vi "read_exist_OPUS.vi"() -> ()   [LabVIEW 2010]
panel:
  in  "functionpath":path=path "D:/Research_CfA/FTS"
  out "used time":dbl
  in  "ifg_path":path=path "D:/Research_CfA/FTS/ha_20150807_ifg"
  in  "spec_path":path=path "D:/Research_CfA/FTS/ha_20150807"
  out "XY Graph 6":cluster{"spec":dbl[], "spec":dbl[]}(graph)
  out "XY Graph 5":cluster{"spec":dbl[], "spec":dbl[]}(graph)
  out "XY Graph 4":cluster{"spec":dbl[], "spec":dbl[]}(graph)
  out "XY Graph 3":cluster{"spec":dbl[], "spec":dbl[]}(graph)
  out "XY Graph 2":cluster{"spec":dbl[], "spec":dbl[]}(graph)
  out "XY Graph":cluster{"spec":dbl[], "spec":dbl[]}(graph)
  in  "observation":string="ha"
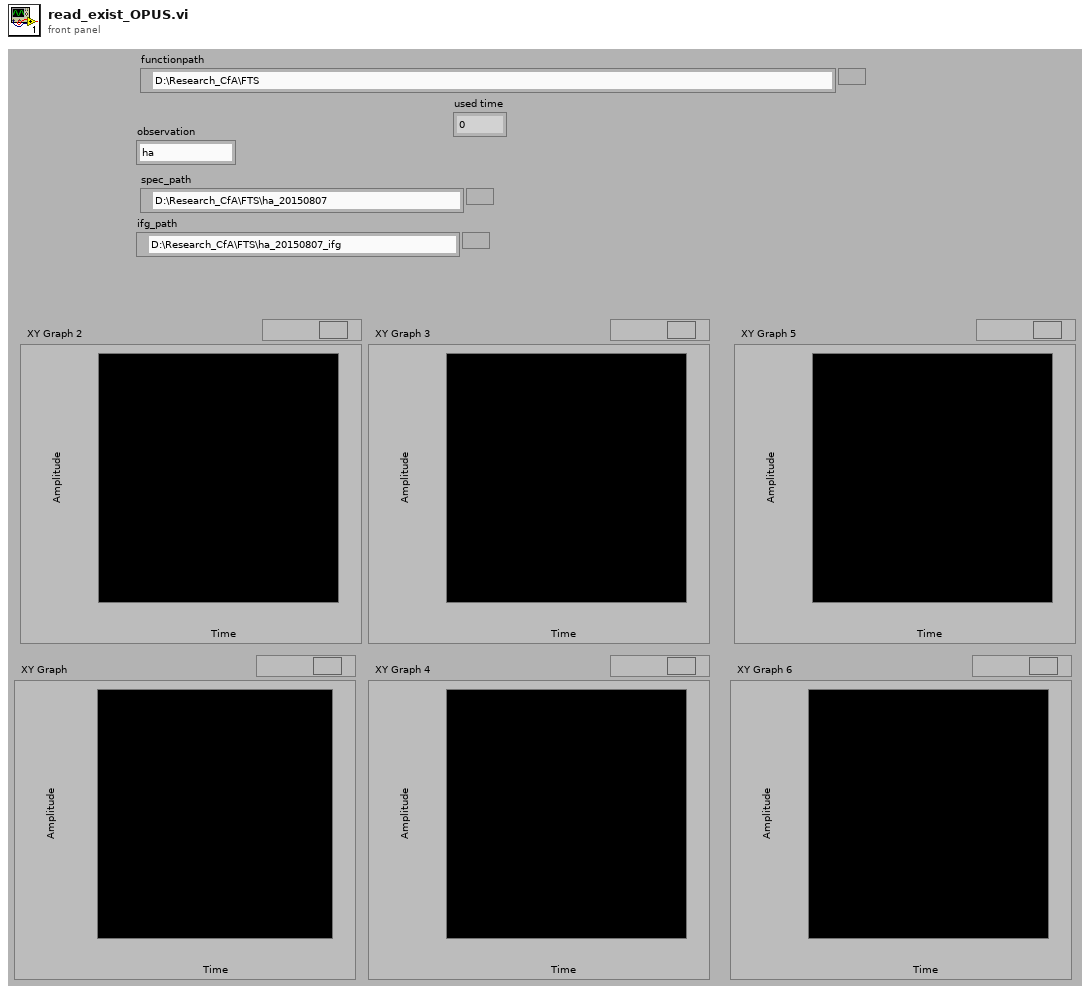
[diagram p1: front panel]
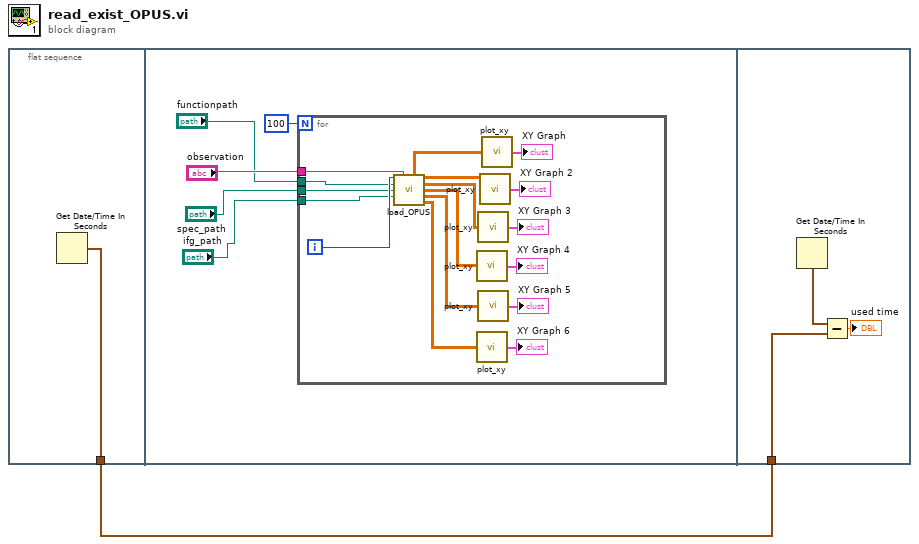
[diagram p0: block diagram]
diagram:
  n1 = flat-sequence {
    tunnel: [w2] -> w1
    tunnel: w1 -> [w26]
    frame #0 {
      n2 = Get Date/Time In Seconds() -> (seconds since 1Jan1904=w2:timestamp)
    }
    frame #1 {
      n3 = for {
        N: 100 -> [_]
        tunnel: "observation" -> [w23]
        tunnel: "spec_path" -> [w16]
        tunnel: "ifg_path" -> [w15]
        tunnel: "functionpath" -> [w14]
        i -> [w24]
        n4 = call "load_OPUS.vi"("fileN"=w24, "observation"=w23, "functionpath"=w14, "spec_path"=w16, "ifg_path"=w15) -> ("spec"=w22:dbl[][], "O2_spec"=w21:dbl[][], "CO2_spec1"=w20:dbl[][], "CO2_spec2"=w19:dbl[][], "CH4_spec1"=w18:dbl[][], "CH4_spec2"=w17:dbl[][])  [unwired: 4 in, 1 out]
        n5 = call "plot_xy.vi"("spec"=w19) -> ("XY Graph"=→"XY Graph 4":cluster{"spec":dbl[], "spec":dbl[]})
        n6 = call "plot_xy.vi"("spec"=w17) -> ("XY Graph"=→"XY Graph 6":cluster{"spec":dbl[], "spec":dbl[]})
        n7 = call "plot_xy.vi"("spec"=w20) -> ("XY Graph"=→"XY Graph 3":cluster{"spec":dbl[], "spec":dbl[]})
        n8 = call "plot_xy.vi"("spec"=w18) -> ("XY Graph"=→"XY Graph 5":cluster{"spec":dbl[], "spec":dbl[]})
        n9 = call "plot_xy.vi"("spec"=w21) -> ("XY Graph"=→"XY Graph 2":cluster{"spec":dbl[], "spec":dbl[]})
        n10 = call "plot_xy.vi"("spec"=w22) -> ("XY Graph"=→"XY Graph":cluster{"spec":dbl[], "spec":dbl[]})
      }
    }
    frame #2 {
      n11 = Get Date/Time In Seconds() -> (seconds since 1Jan1904=w27:timestamp)
      n12 = Subtract(x=w27, y=w26) -> (x-y=→"used time":dbl)
    }
  }
